vi "Initial position.vi"(8 "error in (no error)":errorcluster, 11 "Double Scanner in":refnum<class "Double Scanner.lvclass">) -> (0 "error out":errorcluster, 2 "Initial positions":dbl[](array[numeric]), 3 "Double Scanner out":refnum<class "Double Scanner.lvclass">)   [LabVIEW 2017, in "Double Scanner.lvclass"]
uses:
  Double Scanner.lvclass
  Scanner/Scanner.lvclass
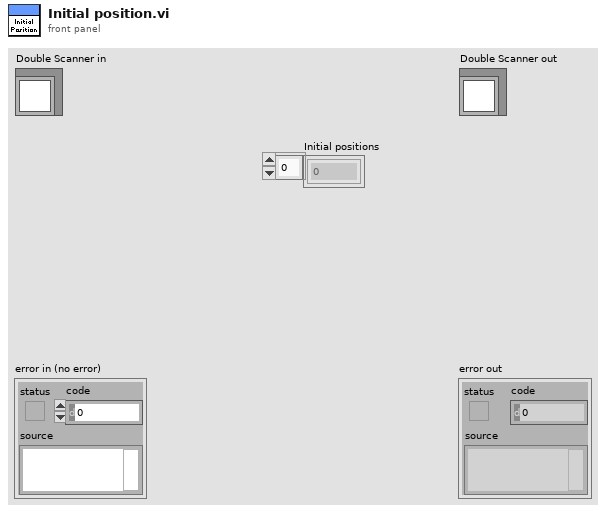
[diagram p1: front panel]
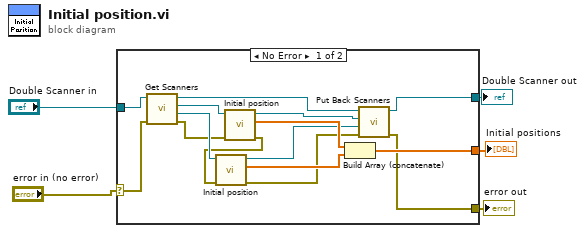
[diagram p0: block diagram]
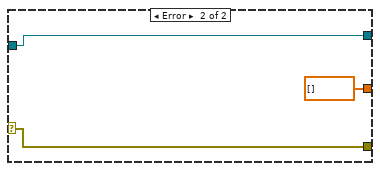
[diagram p2: hidden frame]
diagram:
  n1 = case shown="No Error" "error in (no error)" {
    selector: "error in (no error)" -> [w19 w22]
    tunnel: "Double Scanner in" -> [w20 w23]
    tunnel: [w6 w22] -> w3
    tunnel: [w8 w23] -> w2
    tunnel: [w14 dbl[] []] -> w1
    frame No Error {
      n2 = call-dynamic "Get Scanners.vi"("error in (no error)"=w19, "Double Scanner in"=w20) -> ("error out"=w16:errorcluster, "Scanner 2 out"=w17:refnum<class "Scanner.lvclass">, "Scanner 1 out"=w18:refnum<class "Scanner.lvclass">, "Double Scanner out"=w11:refnum<class "Double Scanner.lvclass">)  [unwired: 6 in]
      n3 = call-dynamic "Initial position.vi"("error in (no error)"=w16, "Scanner in"=w18) -> ("error out"=w15:errorcluster, "Initial positions"=w12:dbl[], "Scanner out"=w10:refnum<class "Scanner.lvclass">)  [unwired: 7 in]
      n4 = call-dynamic "Initial position.vi"("error in (no error)"=w15, "Scanner in"=w17) -> ("error out"=w7:errorcluster, "Initial positions"=w13:dbl[], "Scanner out"=w9:refnum<class "Scanner.lvclass">)  [unwired: 7 in]
      n5 = Build Array (concatenate)(w12, w13) -> (w14:dbl[])
      n6 = call-dynamic "Put Back Scanners.vi"("error in (no error)"=w7, "Scanner 2 in"=w9, "Scanner 1 in"=w10, "Double Scanner in"=w11) -> ("error out"=w6:errorcluster, "Double Scanner out"=w8:refnum<class "Double Scanner.lvclass">)  [unwired: 6 in]
    }
    frame Error {
    }
  }
  "error out" <- w3
  "Double Scanner out" <- w2
  "Initial positions" <- w1
